vi "example_GCommand.vi"() -> ()   [LabVIEW 2021]
uses:
  <vilib>/Galil/resources/gclib/gclib.lvlib
panel:
  out "Error Out":errorcluster
  in  "IP Address":string="192.168.1.77"
  out "Response":string="\r\n:"
  in  "Command":string="MG TIME"
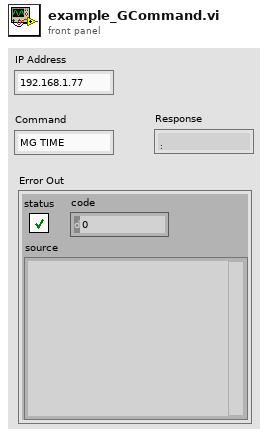
[diagram p1: front panel]
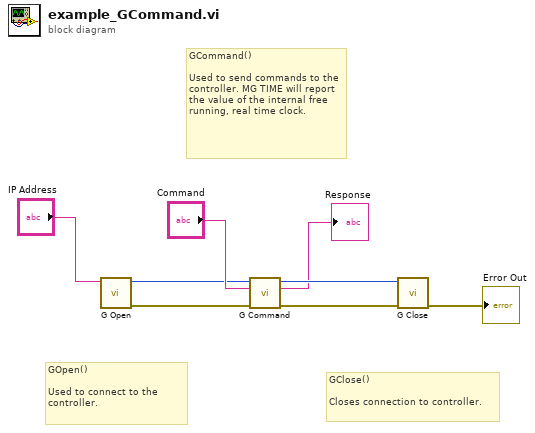
[diagram p0: block diagram]
diagram:
  # "GClose()\n\nCloses connection to controller."
  # "GCommand()\n\nUsed to send commands to the controller. MG TIME will report the value of the internal free running, real time clock."
  # "GOpen()\n\nUsed to connect to the controller."
  n1 = call <vilib>:"G Open.vi"("address"="IP Address") -> ("error out"=w1:errorcluster, "g out"=w3:u64)  [unwired: 8 in]
  n2 = call <vilib>:"G Command.vi"("g"=w3, "command"="Command", "error in (no error)"=w1) -> ("g out"=w8:u64, "buffer out"=→"Response":string, "error out"=w5:errorcluster)  [unwired: 10 in]
  n3 = call <vilib>:"G Close.vi"("error in (no error)"=w5, "g"=w8) -> ("error out"=→"Error Out":errorcluster)  [unwired: 9 in]
